vi "FuncImg-Close UI refs.vi"   [LabVIEW 2013]
uses:
  Global variables/gl_Functional Imaging-Global variables.vi
types:
  T1 = typedef "Functional Imging UI Refs.ctl" = cluster{"Menu ref":refnum<k9>, "Image control":refnum<vi>, "VI ref":refnum<vi>, "XGrapher":refnum<vi>, "Smoothing":refnum<vi>, "POI Averaging":refnum<vi>, "Normalize":refnum<vi>, "POI data points in each trial":refnum<vi>, "Channel":refnum<vi>, "Experiment data folder path":refnum<vi>, "[ROI vis]":refnum<vi>, "[Groups] visbl":T2, "Group Name":refnum<vi>, "POI index":refnum<vi>, "Trial No.":refnum<vi>, "Intensity Zoom":refnum<vi>, "Trial Cursor Enabled":refnum<vi>, "Number of Trials (ind 1)":refnum<vi>, "Number of Trials (ind 2)":refnum<vi>, "MiniScans Available":refnum<vi>, "POI Available":refnum<vi>, "Defer graph updates":refnum<vi>, "Waveform selector":refnum<vi>, "#of selected POI":refnum<vi>, "#of selected MiniScans":refnum<vi>, "#of selected groups":refnum<vi>, "Max Z-Projection":refnum<vi>, "Z-Plane Selector":refnum<vi>, "Index of miniscan point to visualise":refnum<vi>, "ROI vis. mode":refnum<vi>, "Total # of points":refnum<vi>, "Index of group clicked on":refnum<vi>, "Pane 1":refnum<vi>, "Pane 2":refnum<vi>, "Pane 3":refnum<vi>, "Pane 4":refnum<vi>, "Pane 5":refnum<vi>, "Pane 6":refnum<vi>, "Deselect all ROI":refnum<vi>, "Deselect all groups":refnum<vi>}
  T2 = typedef "Groups array referecne.ctl" = refnum<vi>
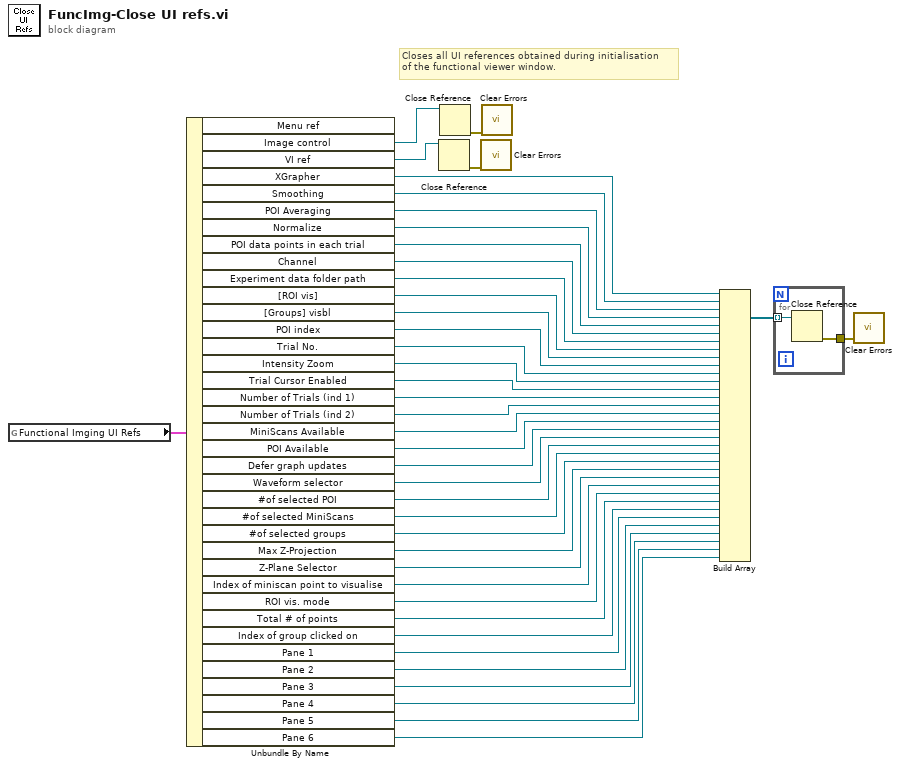
[diagram p0: block diagram]
diagram:
  # "Closes all UI references obtained during initialisation\nof the functional viewer window."
  n1 = global read "gl_Functional Imaging-Global variables.vi" "Functional Imging UI Refs"() -> (w39:T1)
  n2 = Unbundle By Name(w39) -> ("Image control"=w9:refnum<vi>, "VI ref"=w7:refnum<vi>, "XGrapher"=w16:refnum<vi>, "Smoothing"=w15:refnum<vi>, "POI Averaging"=w14:refnum<vi>, "Normalize"=w13:refnum<vi>, "POI data points in each trial"=w17:refnum<vi>, "Channel"=w18:refnum<vi>, "Experiment data folder path"=w19:refnum<vi>, "[ROI vis]"=w20:refnum<vi>, "[Groups] visbl"=w21:T2, "POI index"=w22:refnum<vi>, "Trial No."=w23:refnum<vi>, "Intensity Zoom"=w24:refnum<vi>, "Trial Cursor Enabled"=w25:refnum<vi>, "Number of Trials (ind 1)"=w27:refnum<vi>, "Number of Trials (ind 2)"=w26:refnum<vi>, "MiniScans Available"=w28:refnum<vi>, "POI Available"=w29:refnum<vi>, "Defer graph updates"=w30:refnum<vi>, "Waveform selector"=w31:refnum<vi>, "#of selected POI"=w32:refnum<vi>, "#of selected MiniScans"=w33:refnum<vi>, "#of selected groups"=w34:refnum<vi>, "Max Z-Projection"=w35:refnum<vi>, "Z-Plane Selector"=w37:refnum<vi>, "Index of miniscan point to visualise"=w38:refnum<vi>, "ROI vis. mode"=w40:refnum<vi>, "Total # of points"=w41:refnum<vi>, "Index of group clicked on"=w10:refnum<vi>, "Pane 1"=w6:refnum<vi>, "Pane 2"=w5:refnum<vi>, "Pane 3"=w4:refnum<vi>, "Pane 4"=w3:refnum<vi>, "Pane 5"=w2:refnum<vi>, "Pane 6"=w1:refnum<vi>)  [unwired: 1 out]
  n3 = Close Reference(reference=w7) -> (error out=w8:errorcluster)  [unwired: 1 in]
  n4 = Close Reference(reference=w9) -> (error out=w36:errorcluster)  [unwired: 1 in]
  n5 = call <vilib>:"Clear Errors.vi"("error in (no error)"=w8) -> ()  [unwired: 6 in, 1 out]
  n6 = call <vilib>:"Clear Errors.vi"("error in (no error)"=w36) -> ()  [unwired: 6 in, 1 out]
  n7 = Build Array(w16, w15, w14, w13, w17, w18, w19, w20, w21, w22, w23, w24, w25, w27, w26, w28, w29, w30, w31, w32, w33, w34, w35, w37, w38, w40, w41, w10, w6, w5, w4, w3, w2, w1) -> (w12:refnum<vi>[])
  n8 = for {
    tunnel: w12 -> [w43] mode=indexing
    tunnel: [w42] -> w11
    n9 = Close Reference(reference=w43) -> (error out=w42:errorcluster)  [unwired: 1 in]
  }
  n10 = call <vilib>:"Clear Errors.vi"("error in (no error)"=w11) -> ()  [unwired: 6 in, 1 out]
